vi "Map.vi"() -> (0 "appended array":cluster{"Array":dbl[], "Array 2":dbl[]}[](array[cluster])=[{"Array"=[0.0, 6.0, 6.0, 0.0, 1.0, 1.69, 1.0, 4.99, 4.99, 4.99, 1.0, 1.0, 4.99, 4.39, 4.99], "Array 2"=[0.0, 0.0, 4.0, 4.0, 3.4, 1.2, 1.2, 3.4, 4.0, 0.0, 0.0, 4.0, 1.2, 1.2, 1.0]}, {"Array"=[0.0, 0.0, 6000.0, 6000.0, 0.0], "Array 2"=[0.0, 4000.0, 4000.0, 0.0, 0.0]}, {"Array"=[1000.0, 1000.0, 1090.0, 1090.0, 1000.0], "Array 2"=[0.0, 3400.0, 3400.0, 0.0, 0.0]}, {"Array"=[4990.0, 4990.0, 5080.0, 5080.0, 4990.0], "Array 2"=[1000.0, 3400.0, 3400.0, 1000.0, 1000.0]}, {"Array"=[1690.0, 4390.0, 4390.0, 1690.0, 1690.0], "Array 2"=[1000.0, 1000.0, 1200.0, 1200.0, 1000.0]}, {"Array"=[1690.0, 1690.0, 2190.0, 2190.0, 1690.0], "Array 2"=[2900.0, 3400.0, 3400.0, 2900.0, 2900.0]}, {"Array"=[2790.0, 2790.0, 3290.0, 3290.0, 2790.0], "Array 2"=[2900.0, 3400.0, 3400.0, 2900.0, 2900.0]}, {"Array"=[3890.0, 3890.0, 4390.0, 4390.0, 3890.0], "Array 2"=[2900.0, 3400.0, 3400.0, 2900.0, 2900.0]}, {"Array"=[1690.0, 1690.0, 2190.0, 2190.0, 1690.0], "Array 2"=[1800.0, 2300.0, 2300.0, 1800.0, 1800.0]}, {"Array"=[2790.0, 2790.0, 3290.0, 3290.0, 2790.0], "Array 2"=[1800.0, 2300.0, 2300.0, 1800.0, 1800.0]}, {"Array"=[3890.0, 3890.0, 4390.0, 4390.0, 3890.0], "Array 2"=[1800.0, 2300.0, 2300.0, 1800.0, 1800.0]}, {"Array"=[1690.0, 1690.0, 2190.0, 2190.0, 1690.0], "Array 2"=[1800.0, 2300.0, 2300.0, 1800.0, 1800.0]}, {"Array"=[2790.0, 2790.0, 3290.0, 3290.0, 2790.0], "Array 2"=[1800.0, 2300.0, 2300.0, 1800.0, 1800.0]}, {"Array"=[3890.0, 3890.0, 4390.0, 4390.0, 3890.0], "Array 2"=[1800.0, 2300.0, 2300.0, 1800.0, 1800.0]}, {"Array"=[1690.0, 1690.0, 2190.0, 2190.0, 1690.0], "Array 2"=[1800.0, 2300.0, 2300.0, 1800.0, 1800.0]}, {"Array"=[2790.0, 2790.0, 3290.0, 3290.0, 2790.0], "Array 2"=[1800.0, 2300.0, 2300.0, 1800.0, 1800.0]}, {"Array"=[3890.0, 3890.0, 4390.0, 4390.0, 3890.0], "Array 2"=[1800.0, 2300.0, 2300.0, 1800.0, 1800.0]}, {"Array"=[1690.0, 1690.0, 2190.0, 2190.0, 1690.0], "Array 2"=[1800.0, 2300.0, 2300.0, 1800.0, 1800.0]}, {"Array"=[2790.0, 2790.0, 3290.0, 3290.0, 2790.0], "Array 2"=[1800.0, 2300.0, 2300.0, 1800.0, 1800.0]}, {"Array"=[3890.0, 3890.0, 4390.0, 4390.0, 3890.0], "Array 2"=[1800.0, 2300.0, 2300.0, 1800.0, 1800.0]}, {"Array"=[1690.0, 1690.0, 2190.0, 2190.0, 1690.0], "Array 2"=[1800.0, 2300.0, 2300.0, 1800.0, 1800.0]}, {"Array"=[2790.0, 2790.0, 3290.0, 3290.0, 2790.0], "Array 2"=[1800.0, 2300.0, 2300.0, 1800.0, 1800.0]}, {"Array"=[3890.0, 3890.0, 4390.0, 4390.0, 3890.0], "Array 2"=[1800.0, 2300.0, 2300.0, 1800.0, 1800.0]}])   [LabVIEW 2016]
panel:
  in  "building 2":cluster{"Array":dbl[], "Array 2":dbl[]}={"Array"=[1690.0, 1690.0, 2190.0, 2190.0, 1690.0], "Array 2"=[2900.0, 3400.0, 3400.0, 2900.0, 2900.0]}
  in  "grass":cluster{"Array":dbl[], "Array 2":dbl[]}={"Array"=[1690.0, 4390.0, 4390.0, 1690.0, 1690.0], "Array 2"=[1000.0, 1000.0, 1200.0, 1200.0, 1000.0]}
  in  "wall 2":cluster{"Array":dbl[], "Array 2":dbl[]}={"Array"=[4990.0, 4990.0, 5080.0, 5080.0, 4990.0], "Array 2"=[1000.0, 3400.0, 3400.0, 1000.0, 1000.0]}
  in  "wall 1":cluster{"Array":dbl[], "Array 2":dbl[]}={"Array"=[1000.0, 1000.0, 1090.0, 1090.0, 1000.0], "Array 2"=[0.0, 3400.0, 3400.0, 0.0, 0.0]}
  in  "building":cluster{"Array":dbl[], "Array 2":dbl[]}={"Array"=[1690.0, 1690.0, 2190.0, 2190.0, 1690.0], "Array 2"=[2900.0, 3400.0, 3400.0, 2900.0, 2900.0]}
  in  "border":cluster{"Array":dbl[], "Array 2":dbl[]}={"Array"=[0.0, 0.0, 6000.0, 6000.0, 0.0], "Array 2"=[0.0, 4000.0, 4000.0, 0.0, 0.0]}
  out "XY Graph":cluster{dbl[], dbl[]}[](graph)=[{[0.0, 6.0, 6.0, 0.0, 1.0, 1.69, 1.0, 4.99, 4.99, 4.99, 1.0, 1.0, 4.99, 4.39, 4.99], [0.0, 0.0, 4.0, 4.0, 3.4, 1.2, 1.2, 3.4, 4.0, 0.0, 0.0, 4.0, 1.2, 1.2, 1.0]}, {[0.0, 0.0, 6000.0, 6000.0, 0.0], [0.0, 4000.0, 4000.0, 0.0, 0.0]}, {[1000.0, 1000.0, 1090.0, 1090.0, 1000.0], [0.0, 3400.0, 3400.0, 0.0, 0.0]}, {[4990.0, 4990.0, 5080.0, 5080.0, 4990.0], [1000.0, 3400.0, 3400.0, 1000.0, 1000.0]}, {[1690.0, 4390.0, 4390.0, 1690.0, 1690.0], [1000.0, 1000.0, 1200.0, 1200.0, 1000.0]}, {[1690.0, 1690.0, 2190.0, 2190.0, 1690.0], [2900.0, 3400.0, 3400.0, 2900.0, 2900.0]}, {[2790.0, 2790.0, 3290.0, 3290.0, 2790.0], [2900.0, 3400.0, 3400.0, 2900.0, 2900.0]}, {[3890.0, 3890.0, 4390.0, 4390.0, 3890.0], [2900.0, 3400.0, 3400.0, 2900.0, 2900.0]}, {[1690.0, 1690.0, 2190.0, 2190.0, 1690.0], [1800.0, 2300.0, 2300.0, 1800.0, 1800.0]}, {[2790.0, 2790.0, 3290.0, 3290.0, 2790.0], [1800.0, 2300.0, 2300.0, 1800.0, 1800.0]}, {[3890.0, 3890.0, 4390.0, 4390.0, 3890.0], [1800.0, 2300.0, 2300.0, 1800.0, 1800.0]}, {[1690.0, 1690.0, 2190.0, 2190.0, 1690.0], [1800.0, 2300.0, 2300.0, 1800.0, 1800.0]}, {[2790.0, 2790.0, 3290.0, 3290.0, 2790.0], [1800.0, 2300.0, 2300.0, 1800.0, 1800.0]}, {[3890.0, 3890.0, 4390.0, 4390.0, 3890.0], [1800.0, 2300.0, 2300.0, 1800.0, 1800.0]}, {[1690.0, 1690.0, 2190.0, 2190.0, 1690.0], [1800.0, 2300.0, 2300.0, 1800.0, 1800.0]}, {[2790.0, 2790.0, 3290.0, 3290.0, 2790.0], [1800.0, 2300.0, 2300.0, 1800.0, 1800.0]}, {[3890.0, 3890.0, 4390.0, 4390.0, 3890.0], [1800.0, 2300.0, 2300.0, 1800.0, 1800.0]}, {[1690.0, 1690.0, 2190.0, 2190.0, 1690.0], [1800.0, 2300.0, 2300.0, 1800.0, 1800.0]}, {[2790.0, 2790.0, 3290.0, 3290.0, 2790.0], [1800.0, 2300.0, 2300.0, 1800.0, 1800.0]}, {[3890.0, 3890.0, 4390.0, 4390.0, 3890.0], [1800.0, 2300.0, 2300.0, 1800.0, 1800.0]}, {[1690.0, 1690.0, 2190.0, 2190.0, 1690.0], [1800.0, 2300.0, 2300.0, 1800.0, 1800.0]}, {[2790.0, 2790.0, 3290.0, 3290.0, 2790.0], [1800.0, 2300.0, 2300.0, 1800.0, 1800.0]}, {[3890.0, 3890.0, 4390.0, 4390.0, 3890.0], [1800.0, 2300.0, 2300.0, 1800.0, 1800.0]}]
  in  "Map":cluster{"X\nX":dbl, "Y":dbl}[](array[cluster])=[{"X\nX"=0.0, "Y"=0.0}, {"X\nX"=6.0, "Y"=0.0}, {"X\nX"=6.0, "Y"=4.0}, {"X\nX"=0.0, "Y"=4.0}, {"X\nX"=1.0, "Y"=3.4}, {"X\nX"=1.69, "Y"=1.2}, {"X\nX"=1000.0, "Y"=1200.0}, {"X\nX"=4.99, "Y"=3.4}, {"X\nX"=4.99, "Y"=4.0}, {"X\nX"=4.99, "Y"=0.0}, {"X\nX"=1.0, "Y"=0.0}, {"X\nX"=1.0, "Y"=4.0}, {"X\nX"=4.99, "Y"=1.2}, {"X\nX"=4.39, "Y"=1.2}, {"X\nX"=4.99, "Y"=1.0}]
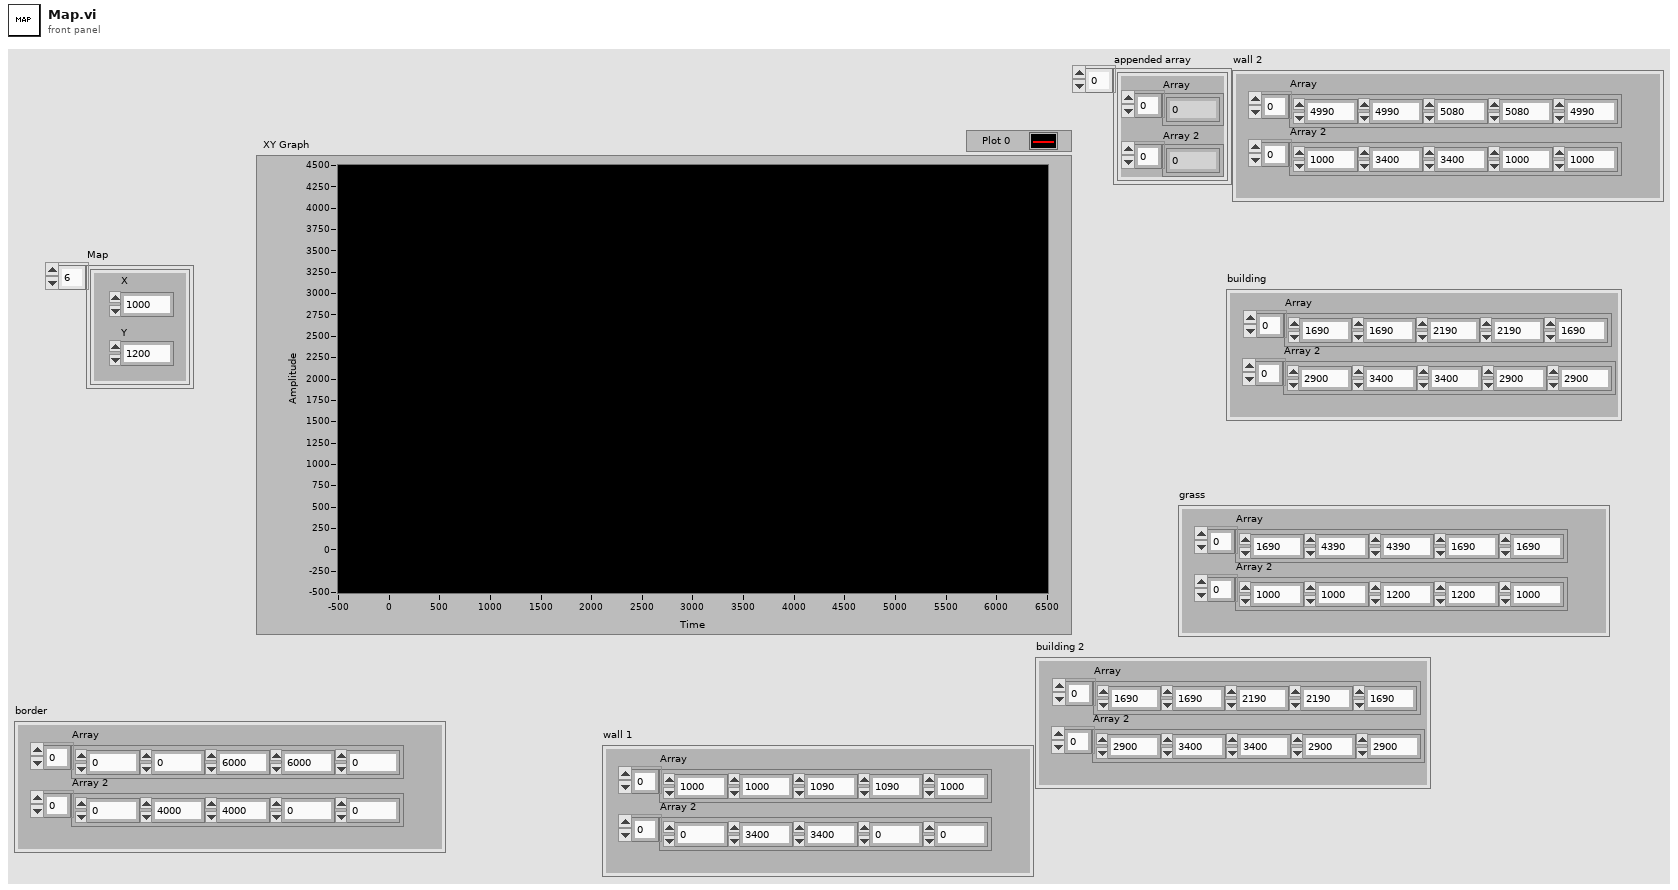
[diagram p1: front panel]
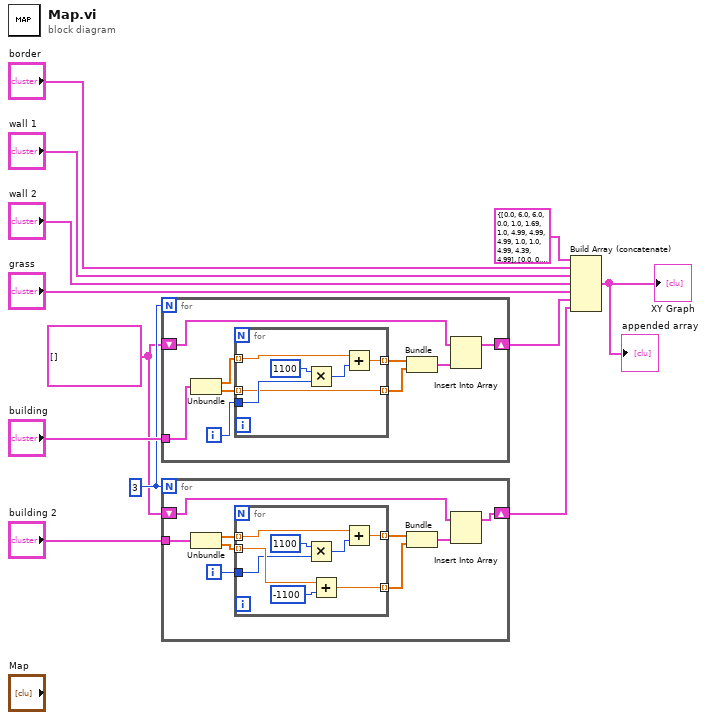
[diagram p0: block diagram]
diagram:
  w1 = cluster{dbl[], dbl[]}[] []
  w3 = 3
  n1 = for {
    N: w3 -> [_]
    shift-right: [w16] -> w6
    shift-left: w1 -> [w15]
    tunnel: "building" -> [w13]
    i -> [w19]
    n2 = Unbundle(w13) -> ("Array"=w21:dbl[], "Array 2"=w20:dbl[])
    n3 = for {
      tunnel: w21 -> [w27] mode=indexing
      tunnel: w20 -> [w22] mode=indexing
      tunnel: w19 -> [w24]
      tunnel: [w23] -> w18 mode=indexing
      tunnel: [w22] -> w17 mode=indexing
      n4 = Multiply(x=1100, y=w24) -> (x*y=w26:i32)
      n5 = Add(x=w27, y=w26) -> (x+y=w23:dbl)
    }
    n6 = Bundle(w18, w17) -> (w14:cluster{dbl[], dbl[]})  [unwired: 1 in]
    n7 = Insert Into Array(array=w15, new element=w14) -> (w16:cluster{dbl[], dbl[]}[])  [unwired: 1 in]
  }
  n8 = for {
    N: w3 -> [_]
    shift-right: [w31] -> w4
    shift-left: w1 -> [w30]
    tunnel: "building 2" -> [w28]
    i -> [w34]
    n9 = Unbundle(w28) -> ("Array"=w36:dbl[], "Array 2"=w35:dbl[])
    n10 = for {
      tunnel: w36 -> [w44] mode=indexing
      tunnel: w35 -> [w43] mode=indexing
      tunnel: w34 -> [w40]
      tunnel: [w39] -> w33 mode=indexing
      tunnel: [w38] -> w32 mode=indexing
      n11 = Multiply(x=1100, y=w40) -> (x*y=w42:i32)
      n12 = Add(x=w43, y=-1100 ("x")) -> (x+y=w38:dbl)
      n13 = Add(x=w44, y=w42) -> (x+y=w39:dbl)
    }
    n14 = Bundle(w33, w32) -> (w29:cluster{dbl[], dbl[]})  [unwired: 1 in]
    n15 = Insert Into Array(array=w30, new element=w29) -> (w31:cluster{dbl[], dbl[]}[])  [unwired: 1 in]
  }
  n16 = Build Array (concatenate)(cluster{dbl[], dbl[]} {[0.0, 6.0, 6.0, 0.0, 1.0, 1.69, 1.0, 4.99, 4.99, 4.99, 1.0, 1.0, 4.99, 4.39, 4.99], [0.0, 0.0, 4.0, 4.0, 3.4, 1.2, 1.2, 3.4, 4.0, 0.0, 0.0, 4.0, 1.2, 1.2, 1.0]} ("output cluster"), "border", "wall 1", "wall 2", "grass", w6, w4) -> (→"XY Graph" →"appended array":cluster{"Array":dbl[], "Array 2":dbl[]}[])
